vi "rep_cap_reset.vi"(7 "Rep Cap Name":string, 8 "error in":errorcluster, 9 "Repeated Capabilities":T1(array[cluster]), 11 "VISA resource name":refnum<visa-resource-name>) -> (0 "error out":errorcluster, 3 "VISA resource name out":refnum<visa-resource-name>)   [LabVIEW 2014, in "rszvl_rsidr_core.lvlib"]
uses:
  rszvl_rsidr_core.lvlib
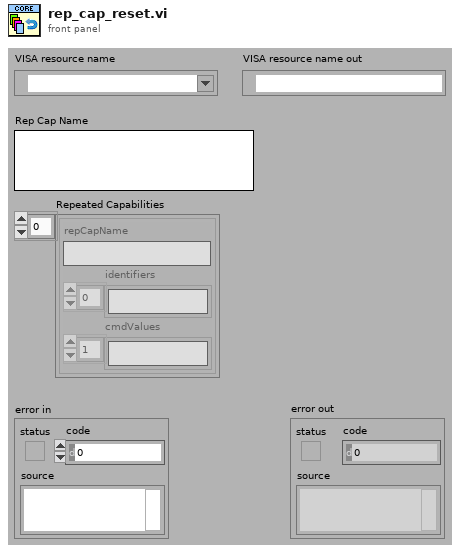
[diagram p1: front panel]
types:
  T1 = cluster{"repCapName":string, "identifiers":string[], "cmdValues":string[]}[]
  T2 = enum16{"Initialize", "Get Cmd Value", "Reset Rep Cap", "Add Rep Cap", "Remove Rep Cap", "Get Rep Cap ID range", "Get Count", "Clear", "Find Name from NameID", "Get First NameID"}
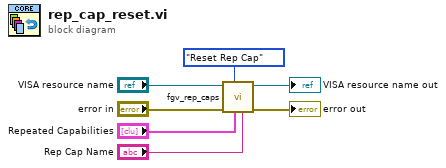
[diagram p0: block diagram]
diagram:
  n1 = call "fgv_rep_caps.vi"("RepCapName in (\"\")"="Rep Cap Name", "Repeated Capabilities (Empty)"="Repeated Capabilities", "Operation"=T2."Reset Rep Cap", "error in"="error in", "VISA resource name"="VISA resource name") -> ("error out"=→"error out":errorcluster, "VISA resource name out"=→"VISA resource name out":refnum<visa-resource-name>)  [unwired: 3 in, 2 out]
